vi "子VI-计算Z值.vi"(8 "分层测量结果":dbl[][](array[numeric])) -> (1 "初始化的数组":dbl[][](array[numeric]))   [LabVIEW 2018]
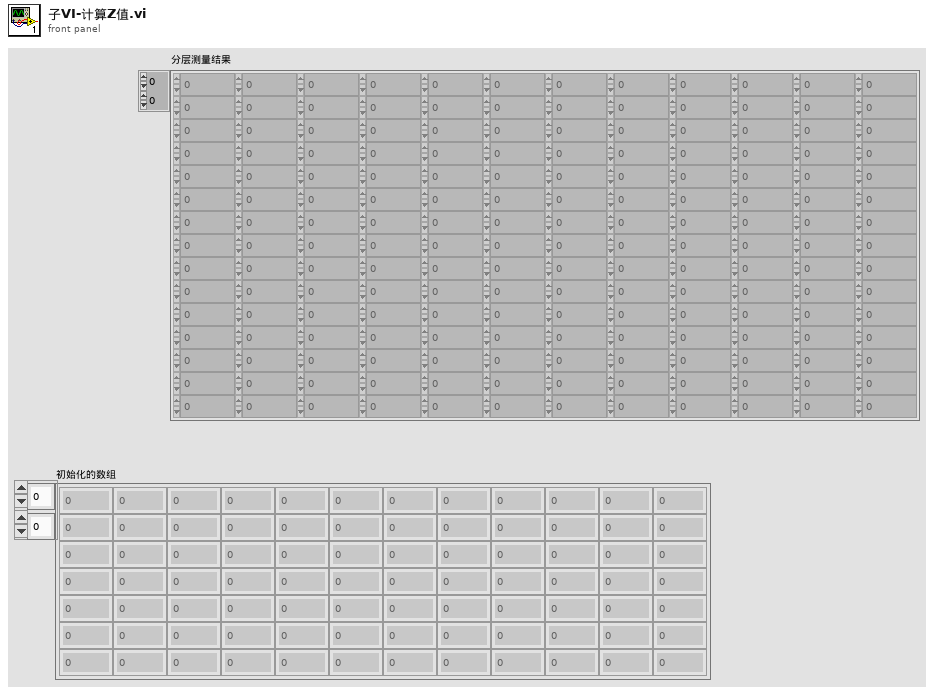
[diagram p1: front panel]
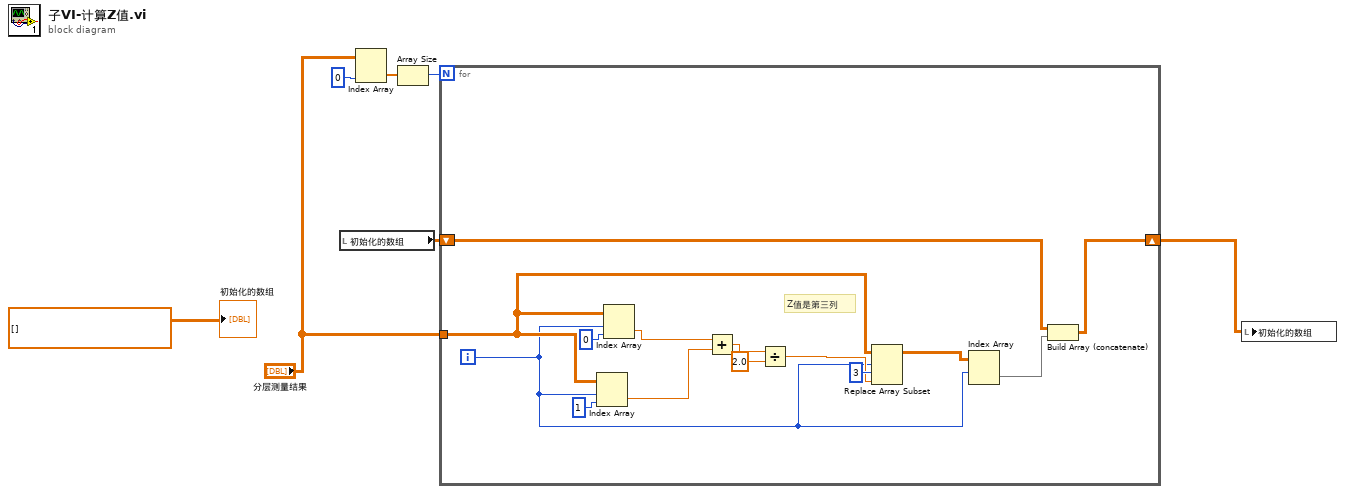
[diagram p0: block diagram]
diagram:
  n1 = local read "初始化的数组"() -> (w1:dbl[][])
  n2 = Index Array(array="分层测量结果", index (col)=0 ("禁用的索引 (列)")) -> (element=w5:dbl[])  [unwired: 1 in]
  n3 = Array Size(array=w5) -> (size(s)=w6:i32)
  n4 = for {
    N: w6 -> [_]
    tunnel: "分层测量结果" -> [w15]
    shift-right: [w9] -> w3
    shift-left: w1 -> [w8]
    i -> [w11]
    # "Z值是第三列"
    n5 = Index Array(array=w15, index (row)=w11, index (col)=1 ("索引 (列)")) -> (element=w18:dbl)
    n6 = Index Array(array=w15, index (row)=w11, index (col)=0 ("索引 (列)")) -> (element=w19:dbl)
    n7 = Add(x=w19, y=w18) -> (x+y=w17:dbl)
    n8 = Divide(x=w17, y=2.0) -> (x/y=w13:dbl)
    n9 = Replace Array Subset(array=w15, new element=w13, index (row)=w11, index (col)=3 ("禁用的索引 (列)")) -> (w12:dbl[][])
    n10 = Index Array(array=w12, index (row)=w11) -> (element=w10:dbl[])  [unwired: 1 in]
    n11 = Build Array (concatenate)(w8, w10) -> (w9:dbl[][])
  }
  n12 = local write "初始化的数组"(w3) -> ()
  "初始化的数组" <- dbl[][] [] ("初始化的数组")
